vi "AES-Shift-Rows.vi"(10 "Inverse":bool, 11 "Data In":u8[](array[numeric])=[0, 0, 0, 0, 0, 0, 0, 0, 0, 0, 0, 0, 0, 0, 0, 0] format="%.0x") -> (3 "Data Out":u8[](array[numeric]) format="%.0x")   [LabVIEW 2017]
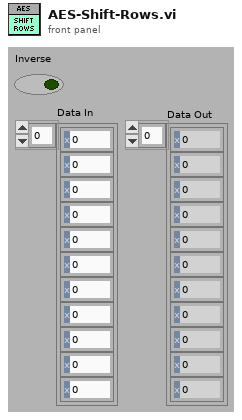
[diagram p1: front panel]
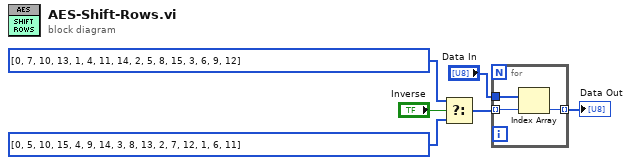
[diagram p0: block diagram]
diagram:
  n1 = Select(t=i32[] [0, 7, 10, 13, 1, 4, 11, 14, 2, 5, 8, 15, 3, 6, 9, 12], s="Inverse", f=i32[] [0, 5, 10, 15, 4, 9, 14, 3, 8, 13, 2, 7, 12, 1, 6, 11]) -> (s? t:f=w3:i32[])
  n2 = for {
    tunnel: w3 -> [w8] mode=indexing
    tunnel: "Data In" -> [w9]
    tunnel: [w7] -> w1 mode=indexing
    n3 = Index Array(array=w9, index=w8) -> (element=w7:u8)
  }
  "Data Out" <- w1
